vi "VCS Find Device Communication Settings.vi"(0 "axis in":cluster{"keyHandle":u32, "nodeId":u16}={"keyHandle"=0, "nodeId"=1}, 1 "pDeviceName":string, 2 "pProtocolStackName":string, 3 "pInterfaceName":string, 4 "pPortName":string, 5 "SizeName":u16, 6 "DialogMode":i32(ring) items=["Progress Dialog", "Progress and Confirmation Dialog", "Confirmation Dialog", "No Dialog"], 7 "error in (no error)":errorcluster, 9 "pBaudrate":u32, 11 "pTimeout":u32) -> (19 "pNodeId out":u16, 20 "axis out":cluster{"keyHandle":u32, "nodeId":u16}={"keyHandle"=0, "nodeId"=1}, 21 "pDeviceName out":string, 22 "pProtocolStackName out":string, 23 "pInterfaceName out":string, 24 "pPortName out":string, 25 "pBaudrate out":u32, 26 "pTimeout out":u32, 27 "error out":errorcluster)   [LabVIEW 2019, in "maxonEPOS.lvlib"]
doc: "With function <B>VCS_FindDeviceCommunicationSettings</B> it is possible to search the communication setting parameters."
uses:
  Examples/maxonEPOS.lvlib
  Resources/EposCmd.dll
  Resources/EposCmd64.dll
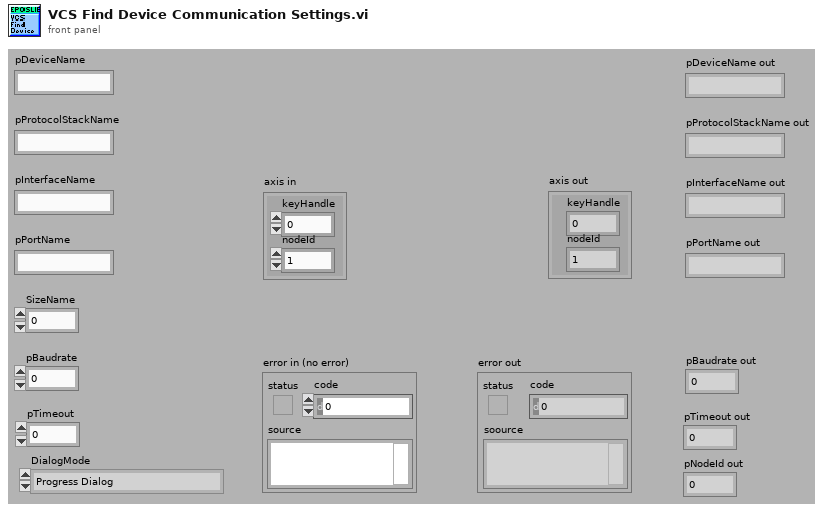
[diagram p1: front panel]
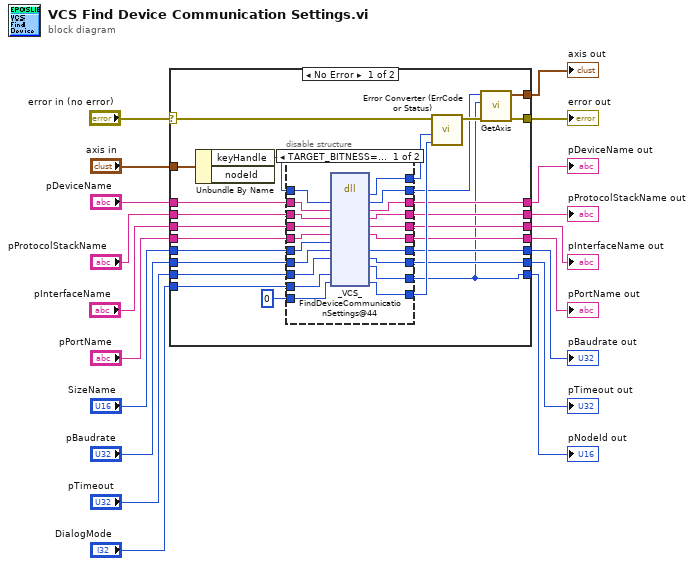
[diagram p0: block diagram]
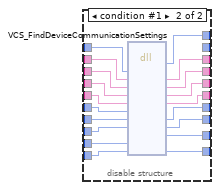
[diagram p2: hidden frame]
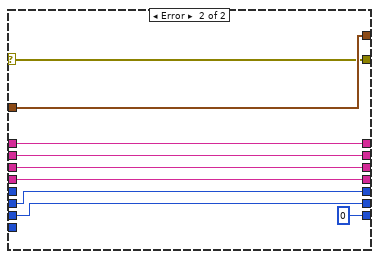
[diagram p3: hidden frame]
diagram:
  n1 = case shown="No Error" "error in (no error)" {
    selector: "error in (no error)" -> [w43 w91]
    tunnel: "axis in" -> [w44 w92]
    tunnel: [w24 w92] -> w18
    tunnel: [w23 w91] -> w17
    tunnel: "pDeviceName" -> [w41 w90]
    tunnel: [w37 w90] -> w14
    tunnel: [w36 w89] -> w13
    tunnel: [w35 w88] -> w12
    tunnel: [w34 w87] -> w11
    tunnel: [w33 w85] -> w10
    tunnel: [w20 u16 0 ("pNodeId")] -> w9
    tunnel: [w32 w86] -> w8
    tunnel: "pProtocolStackName" -> [w31 w89]
    tunnel: "pInterfaceName" -> [w30 w88]
    tunnel: "pPortName" -> [w29 w87]
    tunnel: "SizeName" -> [w28 _]
    tunnel: "pBaudrate" -> [w27 w86]
    tunnel: "pTimeout" -> [w26 w85]
    tunnel: "DialogMode" -> [w25 _]
    frame No Error {
      n2 = Unbundle By Name(w44) -> ("keyHandle"=w40:u32)  [unwired: 1 out]
      n3 = disable-structure shown="TARGET_BITNESS==32, Standard" {
        disable-tunnel: u32 0 ("pErrorCode") -> [w64 w83]
        disable-tunnel: w41 -> [w63 w82]
        disable-tunnel: w40 -> [w62 w81]
        disable-tunnel: [w61 w80] -> w39
        disable-tunnel: [w60 w79] -> w38
        disable-tunnel: [w59 w78] -> w37
        disable-tunnel: [w58 w77] -> w36
        disable-tunnel: [w57 w76] -> w35
        disable-tunnel: [w56 w75] -> w34
        disable-tunnel: [w55 w74] -> w33
        disable-tunnel: [w54 w73] -> w20
        disable-tunnel: [w53 w72] -> w32
        disable-tunnel: w31 -> [w52 w71]
        disable-tunnel: w30 -> [w51 w70]
        disable-tunnel: w29 -> [w50 w69]
        disable-tunnel: w28 -> [w49 w68]
        disable-tunnel: w27 -> [w48 w67]
        disable-tunnel: w26 -> [w47 w66]
        disable-tunnel: w25 -> [w46 w65]
        disable-tunnel: [w45 _] -> w21
        frame condition #0 (active) {
          n4 = dll-call lib="C:/workspace/project/scancon/sw/SSI_Tool/InstrumentsInterfaces/Motordriver/maxon EPOS/Resources/EposCmd.dll" fn="_VCS_FindDeviceCommunicationSettings@44"("pKeyHandle"=w62, "pDeviceName"=w63, "pProtocolStackName"=w52, "pInterfaceName"=w51, "pPortName"=w50, "SizeName"=w49, "pBaudrate"=w48, "pTimeout"=w47, "ShowMsg"=w46, "pErrorCode"=w64) -> (w60:i32, "pKeyHandle"=w45:u32, "pDeviceName"=w59:string, "pProtocolStackName"=w58:string, "pInterfaceName"=w57:string, "pPortName"=w56:string, "pBaudrate"=w53:u32, "pTimeout"=w55:u32, "pNodeId"=w54:u16, "pErrorCode"=w61:u32)  [unwired: 6 in, 2 out]
        }
        frame condition #1 {
          n5 = dll-call lib="C:/LabVIEW/maxon EPOS/Resources/EposCmd64.dll" fn="VCS_FindDeviceCommunicationSettings"("pKeyHandle"=w81, "pDeviceName"=w82, "pProtocolStackName"=w71, "pInterfaceName"=w70, "pPortName"=w69, "SizeName"=w68, "pBaudrate"=w67, "pTimeout"=w66, "ShowMsg"=w65, "pErrorCode"=w83) -> ("return type"=w79:i32, "pDeviceName"=w78:string, "pProtocolStackName"=w77:string, "pInterfaceName"=w76:string, "pPortName"=w75:string, "pBaudrate"=w72:u32, "pTimeout"=w74:u32, "pNodeId"=w73:u16, "pErrorCode"=w80:u32)  [unwired: 7 in, 2 out]
        }
      }
      n6 = call "Error Converter (ErrCode or Status).vi"("error code"=w39, "return type"=w38, "error in (no error)"=w43) -> ("error out"=w22:errorcluster)  [unwired: 7 in]
      n7 = call "GetAxis.vi"("error in (no error)"=w22, "nodeId"=w20, "keyHandle in"=w21) -> ("error out"=w23:errorcluster, "axis out"=w24:cluster{"keyHandle":u32, "nodeId":u16})  [unwired: 7 in]
    }
    frame Error {
    }
  }
  "pDeviceName out" <- w14
  "pProtocolStackName out" <- w13
  "pInterfaceName out" <- w12
  "pPortName out" <- w11
  "pBaudrate out" <- w8
  "pTimeout out" <- w10
  "pNodeId out" <- w9
  "error out" <- w17
  "axis out" <- w18
